vi "CompassIndicatorMerge.vi"() -> ()   [LabVIEW 2017]
uses:
  <vilib>/robotics/Controls/Compass Indicator/Compass Indicator.xctl
panel:
  out "Compass Indicator":dbl(xcontrol)
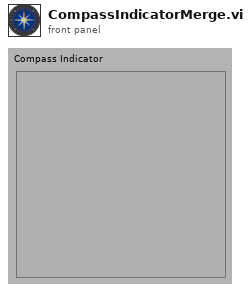
[diagram p1: front panel]
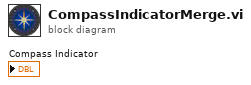
[diagram p0: block diagram]
diagram:
